vi "Win32 Window Handle Wrapper.vi"(8 "error in (no error)":errorcluster, 11 "Win32 Window Handle":i32) -> (0 "error out":errorcluster, 3 "System.Windows.Forms.IWin32Window":refnum<k24>)   [LabVIEW 2020]
doc: "This VI Creates a IWin32Window Typed reference a the Win32 Windows Handle."
uses:
  System.Windows.Forms
  D:/Experiment VIs/Utility VIs/Windows VIs/WindowWrapper.dll
  WindowWrapper.dll
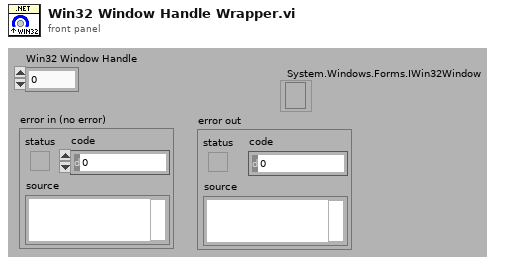
[diagram p1: front panel]
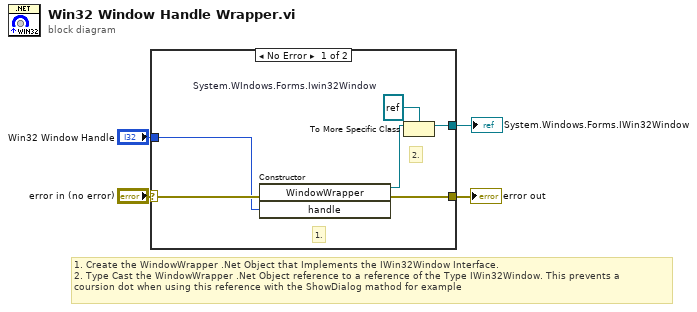
[diagram p0: block diagram]
diagram:
  # "1. Create the WindowWrapper .Net Object that Implements the IWin32Window Interface.\n2. Type Cast the WindowWrapper .Net Object reference to a reference of the Type IWin32Window. This prevents a \ncoursion dot when using this reference with the ShowDialog mathod for example"
  n1 = case shown="No Error" "error in (no error)" {
    selector: "error in (no error)" -> [w8 w11]
    tunnel: "Win32 Window Handle" -> [w7 _]
    tunnel: [w9 w11] -> w3
    tunnel: [w5 _] -> w1
    frame No Error {
      w10 = refnum<k24> refnum  # System.WIndows.Forms.Iwin32Window
      # "2."
      # "1."
      n2 = constructor class="WindowWrapper"(error in=w8, "handle"=w7) -> (reference out=w6:refnum<k24>, error out=w9:errorcluster)  [unwired: 2 in, 2 out]
      n3 = To More Specific Class(target class=w10, reference=w6) -> (specific class reference=w5:refnum<k24>)  [unwired: 1 in, 1 out]
    }
    frame Error {
    }
  }
  "error out" <- w3
  "System.Windows.Forms.IWin32Window" <- w1
